vi "Launcher.vi"   [LabVIEW 2015, in "SCADA Launcher.lvlib"]
doc: "Launcher for the Master Controller SCADA program."
uses:
  SCADA Launcher.lvlib
  Master Controller Core/Master Controller/Master Controller.lvclass
  <vilib>/ActorFramework/Actor/Actor.lvclass
panel:
  # "This is the top launcher of the SCADA Communications application. After running this a seperate window will open that provides the interface to the SCADA application."
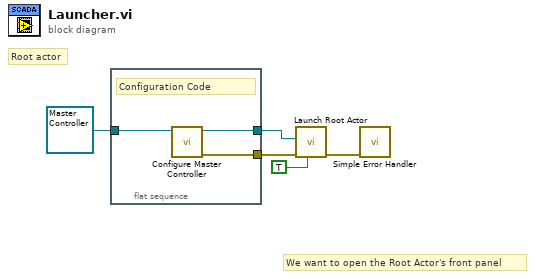
[diagram p0: block diagram]
diagram:
  # "We want to open the Root Actor's front panel"
  # "Root actor"
  n1 = flat-sequence {
    tunnel: refnum<class "Master Controller.lvclass"> refnum ("Master Controller Core.lvlib:Master Controller.lvclass") -> [w8]
    tunnel: [w7] -> w4
    tunnel: [w6] -> w3
    frame #0 {
      # "Configuration Code"
      n2 = call "Configure Master Controller.vi"("Master Controller in"=w8) -> ("error out"=w6:errorcluster, "Master Controller out"=w7:refnum<class "Master Controller.lvclass">)  [unwired: 9 in]
    }
  }
  n3 = call <vilib>:"Launch Root Actor.vi"("Open Actor Core front panel? (F)"=TRUE, "error in (no error)"=w3, "Actor"=w4) -> ("error out"=w1:errorcluster)  [unwired: 7 in, 1 out]
  n4 = call <vilib>:"Simple Error Handler.vi"("error in (no error)"=w1) -> ()  [unwired: 4 in, 5 out]
